vi "ArmPlanToPath.vi"(1 "ArmPlanResponse":T2 {"WristTrajectory"."Time (ms)" items=["TrajectoryDuration_0ms"=0, "TrajectoryDuration_5ms"=5, "TrajectoryDuration_10ms"=10, "TrajectoryDuration_20ms"=20, "TrajectoryDuration_30ms"=30, "TrajectoryDuration_40ms"=40, "TrajectoryDuration_50ms"=50, "TrajectoryDuration_100ms"=100]; "ExtendTrajectory"."Time (ms)" items=["TrajectoryDuration_0ms"=0, "TrajectoryDuration_5ms"=5, "TrajectoryDuration_10ms"=10, "TrajectoryDuration_20ms"=20, "TrajectoryDuration_30ms"=30, "TrajectoryDuration_40ms"=40, "TrajectoryDuration_50ms"=50, "TrajectoryDuration_100ms"=100]; "ShoulderTrajectory"."Time (ms)" items=["TrajectoryDuration_0ms"=0, "TrajectoryDuration_5ms"=5, "TrajectoryDuration_10ms"=10, "TrajectoryDuration_20ms"=20, "TrajectoryDuration_30ms"=30, "TrajectoryDuration_40ms"=40, "TrajectoryDuration_50ms"=50, "TrajectoryDuration_100ms"=100]}) -> (0 "Path":T1[](array[typedef]))   [LabVIEW 2018]
uses:
  TypeDefs/ArmPlanResponse.ctl
  General/MotionProfiling/TypeDefs/TrajectoryPoint.ctl
  <vilib>/Rock Robotics/WPI/ThirdParty/Phoenix-LabVIEW/Motor Controller/Controls/CTRE_Phoenix_MotorControl_TrajectoryPointTimeDur.ctl
  TypeDefs/ArmCoordinate.ctl
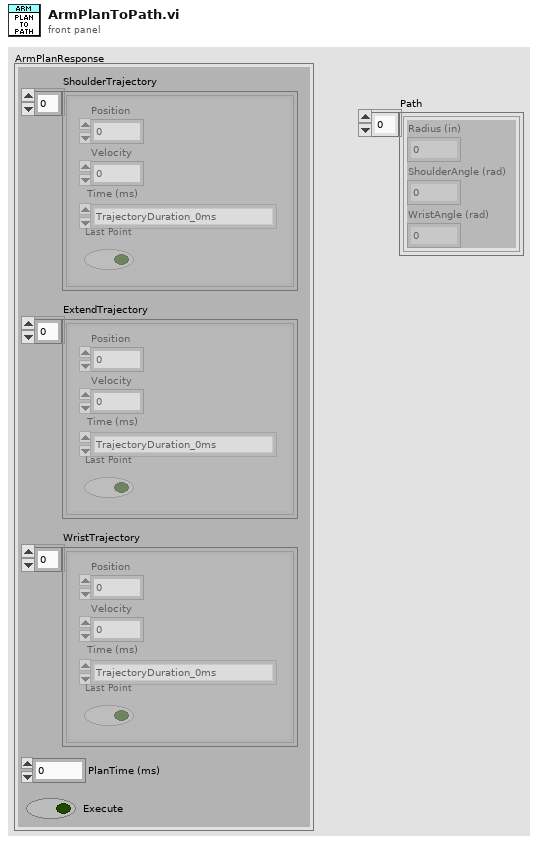
[diagram p1: front panel]
types:
  T1 = typedef "ArmCoordinate.ctl" = cluster{"Radius (in)":dbl, "ShoulderAngle (rad)":dbl, "WristAngle (rad)":dbl}
  T2 = typedef "ArmPlanResponse.ctl" = cluster{"ShoulderTrajectory":T3[], "ExtendTrajectory":T3[], "PlanTime (ms)":u32, "Execute":bool, "WristTrajectory":T3[]}
  T3 = typedef "TrajectoryPoint.ctl" = cluster{"Position ":dbl, "Velocity ":dbl, "Time (ms)":T4, "Last Point":bool}
  T4 = typedef "CTRE_Phoenix_MotorControl_TrajectoryPointTimeDur.ctl" = i32
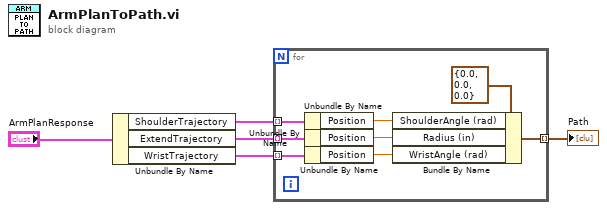
[diagram p0: block diagram]
diagram:
  n1 = Unbundle By Name("ArmPlanResponse") -> ("ShoulderTrajectory"=w4:T3[], "ExtendTrajectory"=w3:T3[], "WristTrajectory"=w2:T3[])
  n2 = for {
    tunnel: w4 -> [w11] mode=indexing
    tunnel: w3 -> [w10] mode=indexing
    tunnel: w2 -> [w9] mode=indexing
    tunnel: [w12] -> w1 mode=indexing
    n3 = Unbundle By Name(w11) -> ("Position"=w8:dbl)
    n4 = Unbundle By Name(w10) -> ("Position"=w7:dbl)
    n5 = Unbundle By Name(w9) -> ("Position"=w6:dbl)
    n6 = Bundle By Name(cluster=T1 {"Radius (in)"=0.0, "ShoulderAngle (rad)"=0.0, "WristAngle (rad)"=0.0} ("Point"), "ShoulderAngle (rad)"=w8, "Radius (in)"=w7, "WristAngle (rad)"=w6) -> (w12:T1)
  }
  "Path" <- w1
